vi "Rapid Voltage Changes.vi"(0 "half-cycle voltage RMS":T1(array[cluster]), 1 "reset? (F)":bool, 5 "RVC settings":T2={"min rate of change [%/s]"=0.5, "steadiness of steady state [%]"=0.2, "min steady state duration [s]"=1.0, "min steady state difference [%]"=0.0, "max voltage change [%]"=3.3}, 7 "voltage flags? (F)":bool[](array[boolean]), 9 "system info in":refnum<class "EP System Info.lvclass">, 11 "error in (no error)":errorcluster) -> (4 "rapid voltage changes events":T4(array[cluster]), 10 "system info out":refnum<class "EP System Info.lvclass">, 15 "error out":errorcluster)   [LabVIEW 2014, in "NI_EP_Power Quality.lvlib"]
doc: "Detects rapid RMS voltage changes between two steady state conditions according to IEC 61000-4-30:2008. The variation in voltage must not exceed the voltage dip threshold, the voltage swell threshold, or the thresholds that contain both voltage dip and voltage swell. EN 50160:2007 defines default threshold values. You also can specify custom threshold values.\n\nThis VI supports measuring single-bus single-line or multiple-bus single-line systems."
uses:
  <vilib>/addons/Electrical Power/PQ/NI_EP_Power Quality.lvlib
  <vilib>/addons/Electrical Power/PQ/Common/Classes/System Info/EP System Info.lvclass
  <vilib>/addons/Electrical Power/PQ/Common/Controls/ep_Phase.ctl
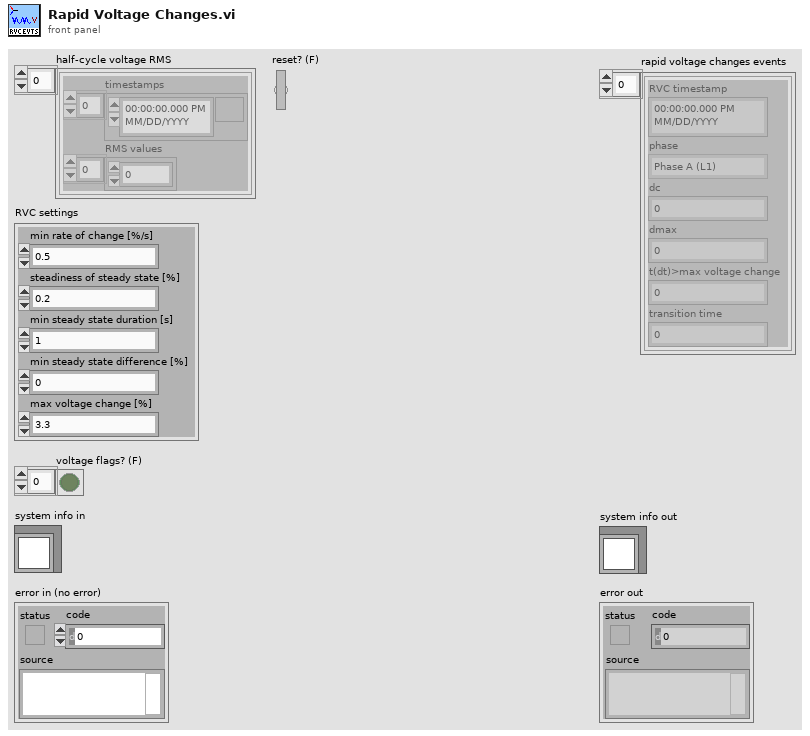
[diagram p1: front panel]
types:
  T1 = cluster{"timestamps":timestamp[], "RMS values":dbl[]}[]
  T2 = cluster{"min rate of change [%/s]":dbl, "steadiness of steady state [%]":dbl, "min steady state duration [s]":dbl, "min steady state difference [%]":dbl, "max voltage change [%]":dbl}
  T3 = typedef "NI_EP_Power Quality.lvlib/ep_Phase.ctl" = enum16{"Phase A (L1)", "Phase B (L2)", "Phase C (L3)", "Phase N", "~3 Phases"}
  T4 = cluster{"RVC timestamp":timestamp, "phase":T3, "dc":dbl, "dmax":dbl, "t(dt)>max voltage change":dbl, "transition time":dbl}[]
  T5 = cluster{"RVC time":timestamp, "phase":T3, "dc":dbl, "dmax":dbl, "t(dt)>max change":dbl, " transition time":dbl}[]
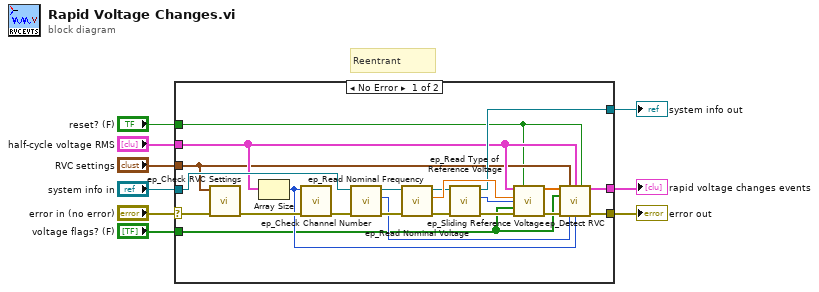
[diagram p0: block diagram]
diagram:
  # "Reentrant"
  n1 = case shown="No Error" "error in (no error)" {
    selector: "error in (no error)" -> [w29 w33]
    tunnel: "system info in" -> [w18 w32]
    tunnel: "reset? (F)" -> [w10 _]
    tunnel: "RVC settings" -> [w14 _]
    tunnel: [w31 _] -> w6
    tunnel: "voltage flags? (F)" -> [w11 _]
    tunnel: "half-cycle voltage RMS" -> [w15 _]
    tunnel: [w17 w32] -> w3
    tunnel: [w30 w33] -> w2
    frame No Error {
      n2 = call <vilib>:"ep_Check RVC Settings.vi"("error in (no error)"=w29, "RVC settings"=w14) -> ("error out"=w20:errorcluster)  [unwired: 9 in]
      n3 = Array Size(array=w15) -> (size(s)=w12:i32)
      n4 = call <vilib>:"ep_Check Channel Number.vi"("channel number"=w12, "error in (no error)"=w20) -> ("error out"=w19:errorcluster)  [unwired: 13 in]
      n5 = call <vilib>:"ep_Read Nominal Frequency.vi"("error in (no error)"=w19, "system info in"=w18) -> ("error out"=w27:errorcluster, "nominal frequency"=w21:enum16{"50 Hz", "60 Hz"}, "system info out"=w28:refnum<class "EP System Info.lvclass">)  [unwired: 6 in, 1 out]
      n6 = call <vilib>:"ep_Read Nominal Voltage.vi"("error in (no error)"=w27, "system info in"=w28) -> ("error out"=w26:errorcluster, "nominal voltage [V]"=w23:dbl, "system info out"=w22:refnum<class "EP System Info.lvclass">)  [unwired: 7 in]
      n7 = call <vilib>:"ep_Read Type of Reference Voltage.vi"("error in (no error)"=w26, "system info in"=w22) -> ("error out"=w25:errorcluster, "type of reference voltage"=w24:enum16{"Constant", "Sliding"}, "system info out"=w17:refnum<class "EP System Info.lvclass">)  [unwired: 7 in]
      n8 = call <vilib>:"ep_Sliding Reference Voltage.vi"("voltage RMS (1/2) (1 cycle)"=w15, "restart (F)"=w10, "nominal voltage [V]"=w23, "type of reference voltage"=w24, "voltage flags"=w11, "error in (no error)"=w25) -> ("reference voltages"=w13:dbl[], "error out"=w16:errorcluster)  [unwired: 8 in]
      n9 = call <vilib>:"ep_Detect RVC.vi"("reference voltages"=w13, "RVC settings"=w14, "half-cycle voltage RMS"=w15, "reset? (F)"=w10, "voltage flags? (F)"=w11, "error in (no error)"=w16, "nominal frequency"=w21, "channel number"=w12) -> ("rapid voltage changes"=w31:T5, "error out"=w30:errorcluster)  [unwired: 6 in]
    }
    frame Error {
    }
  }
  "error out" <- w2
  "rapid voltage changes events" <- w6
  "system info out" <- w3
